vi "To JSON.vi"(6 "Pretty Print?":bool, 8 "error in (no error)":errorcluster, 11 "Double Float in":refnum<class "Abs_Complex Double Float.lvclass">) -> (0 "error out":errorcluster, 2 "JSON":string, 3 "Double Float out":refnum<class "Abs_Complex Double Float.lvclass">)   [LabVIEW 2021, in "Abs_Complex Double Float.lvclass"]
uses:
  Abs_Complex Double Float.lvclass
  C:/Program Files (x86)/National Instruments/LabVIEW 2021/vi.lib/TSA/Abstract Data Classes/Abs_Types/Type/Abs_Type.lvclass
  7e557440-db6b-4515-97f3-062d4c85f86f.vi
  <vilib>/Utility/LVClass/Get LV Class Name.vi
  <vilib>/JDP Science/JSONtext/Variant to JSON Text.vi
  <vilib>/JDP Science/JSONtext/Set Multiple Object Items.vi
  <vilib>/JDP Science/JSONtext/LVClass Serializer/JSONtext LVClass Serializer.lvclass
  Floating Point/Abs_Floating Point.lvclass
  Type/Abs_Type.lvclass
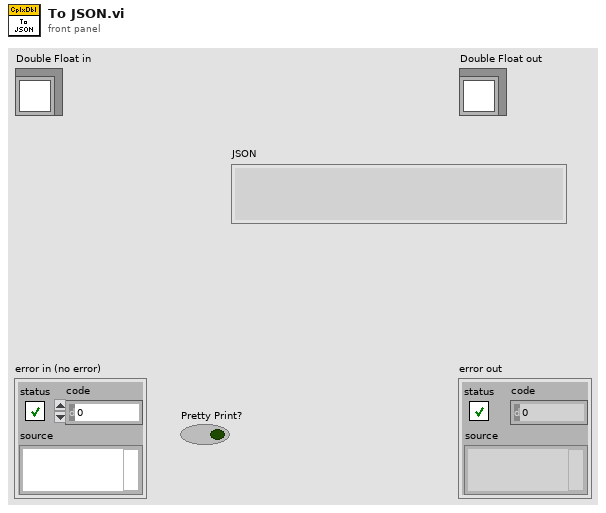
[diagram p1: front panel]
types:
  T1 = typedef "Abs_Complex Double Float.lvclass/Type.ctl" = cdb
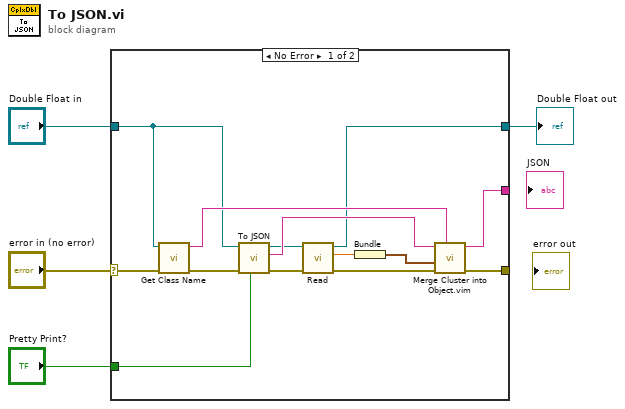
[diagram p0: block diagram]
diagram:
  n1 = case shown="No Error" "error in (no error)" {
    selector: "error in (no error)" -> [w12 w20]
    tunnel: "Double Float in" -> [w6 w19]
    tunnel: [w8 w19] -> w2
    tunnel: [w17 w20] -> _
    tunnel: [w16 _] -> _
    tunnel: "Pretty Print?" -> [w5 _]
    frame No Error {
      n2 = call "Get Class Name.vi"("error in (no error)"=w12, "Abs_Type in"=w6) -> ("error out"=w11:errorcluster, "class name"=w14:string)  [unwired: 8 in]
      n3 = call-parent "To JSON.vi"("Pretty Print?"=w5, "error in (no error)"=w11, "Type in"=w6) -> ("error out"=w10:errorcluster, "JSON"=w13:string, "Type out"=w7:refnum<class "Abs_Complex Double Float.lvclass">)  [unwired: 6 in]
      n4 = call-dynamic "Read.vi"("error in (no error)"=w10, "Double Float.lvclass_340760 in"=w7) -> ("error out"=w9:errorcluster, "Value"=w15:T1, "Double Float.lvclass_340760 out"=w8:refnum<class "Abs_Complex Double Float.lvclass">)  [unwired: 7 in]
      n5 = Bundle("Value"=w15) -> (w18:cluster{"Value":T1})  [unwired: 1 in]
      n6 = call "Merge Cluster into Object.vim"("$Path or Item Name"=w14, "error in (no error)"=w9, "Any Cluster"=w18, "JSON"=w13) -> ("error out"=w17:errorcluster, "<JSON>"=w16:string)  [unwired: 5 in]
    }
    frame Error {
    }
  }
  "Double Float out" <- w2
